vi "Init AC Source.vi"(7 "Trigger frequency  (Hz)":dbl, 8 "error in (no error)":errorcluster, 11 "AC source":T1={"AC Source type"=enum."Agilent 331xxA to 332xxA", "awg lib session"={"type"=enum."Agilent 331xxA to 332xxA", "VISA"="", "enable 10MHz ref"=FALSE, "cmi ckd2"={"VISA"="", "clock source"=enum."Auto", "manual ref clk"=FALSE, "ref clock [Hz]"=0.0, "div mode"=enum."Set divisor directly"}, "cmi sync v3"={"VISA"="", "baud rate [bd/s]"=115200, "source"=enum."Auto", "hv range"=enum."1kV", "fsrc is fixed"=FALSE, "fsrc [Hz]"=10000000.0, "freq integ [s]"=1.0, "freq filter"=5, "trig level"=enum."TTL 5V", "chn1 mode"=enum."Source divider", "chn1 level"=enum."Positive 5V", "chn2 mode"=enum."Source divider", "chn2 level"=enum."Positive 5V", "chn2 div"=1, "chn3 mode"=enum."Chn 1 Active", "chn3 level"=enum."Positive 5V", "chn1 div entry"=enum."Calculate nearest divisor from measured fx", "chn1 dev limit [%]"=1.0, "chn1 check dev"=FALSE}, "trigger"={"source"=enum."Immediate", "level [V]"=0.0, "coupling"=enum."DC", "slope"=enum."POS"}, "HMF2500 cfg"={"Baud Rate"=9600, "Parity"=0, "Data Bits"=8, "Flow Control"=4}}, "DAQmx Device Name"="PXI2Slot6"} {"awg lib session"."HMF2500 cfg"."Flow Control" items=["None", "XON/XOFF", "RTS/CTS", "XON/XOFF & RTS/CTS", "DTR/DSR", "XON/XOFF & DTR/DSR"]; "awg lib session"."HMF2500 cfg"."Data Bits" items=["7"=7, "8"=8]; "awg lib session"."HMF2500 cfg"."Parity" items=["None", "Odd", "Even", "Mark", "Space"]; "awg lib session"."HMF2500 cfg"."Baud Rate" items=["300"=300, "600"=600, "1200"=1200, "2400"=2400, "4800"=4800, "9600"=9600, "19200"=19200]; "awg lib session"."cmi sync v3"."chn2 div" min=1 max=100000000 step=1; "awg lib session"."cmi sync v3"."fsrc [Hz]" format="%_8p"}) -> (0 "error out":errorcluster, 2 "Init status":string, 3 "AC source out":T1={"AC Source type"=enum."Agilent 331xxA to 332xxA", "awg lib session"={"type"=enum."Agilent 331xxA to 332xxA", "VISA"="", "enable 10MHz ref"=FALSE, "cmi ckd2"={"VISA"="", "clock source"=enum."Auto", "manual ref clk"=FALSE, "ref clock [Hz]"=0.0, "div mode"=enum."Set divisor directly"}, "cmi sync v3"={"VISA"="", "baud rate [bd/s]"=115200, "source"=enum."Auto", "hv range"=enum."1kV", "fsrc is fixed"=FALSE, "fsrc [Hz]"=10000000.0, "freq integ [s]"=1.0, "freq filter"=5, "trig level"=enum."TTL 5V", "chn1 mode"=enum."Source divider", "chn1 level"=enum."Positive 5V", "chn2 mode"=enum."Source divider", "chn2 level"=enum."Positive 5V", "chn2 div"=1, "chn3 mode"=enum."Chn 1 Active", "chn3 level"=enum."Positive 5V", "chn1 div entry"=enum."Calculate nearest divisor from measured fx", "chn1 dev limit [%]"=1.0, "chn1 check dev"=FALSE}, "trigger"={"source"=enum."Immediate", "level [V]"=0.0, "coupling"=enum."DC", "slope"=enum."POS"}, "HMF2500 cfg"={"Baud Rate"=9600, "Parity"=0, "Data Bits"=8, "Flow Control"=4}}, "DAQmx Device Name"="PXI2Slot6"} {"awg lib session"."HMF2500 cfg"."Flow Control" items=["None", "XON/XOFF", "RTS/CTS", "XON/XOFF & RTS/CTS", "DTR/DSR", "XON/XOFF & DTR/DSR"]; "awg lib session"."HMF2500 cfg"."Data Bits" items=["7"=7, "8"=8]; "awg lib session"."HMF2500 cfg"."Parity" items=["None", "Odd", "Even", "Mark", "Space"]; "awg lib session"."HMF2500 cfg"."Baud Rate" items=["300"=300, "600"=600, "1200"=1200, "2400"=2400, "4800"=4800, "9600"=9600, "19200"=19200]; "awg lib session"."cmi sync v3"."chn2 div" min=1 max=100000000 step=1; "awg lib session"."cmi sync v3"."fsrc [Hz]" format="%_8p"})   [LabVIEW 2020]
uses:
  Type definitions/AC Source.ctl
  Type definitions/AC Source type.ctl
  external libraries/AWG/AWG Session.ctl
  external libraries/AWG/AWG Type.ctl
  external libraries/AWG/CMI Clock Divider v2/CMI ckd2 Session.ctl
  external libraries/AWG/CMI Clock Divider v2/CMI ckd2 Source Mode.ctl
  external libraries/AWG/CMI Clock Divider v2/CMI ckd2 Divisor Mode.ctl
  external libraries/AWG/CMI Sync V3/CMI Sync V3 session.ctl
  external libraries/AWG/CMI Sync V3/Configure/CMI Sync V3 Reference Clock Source.ctl
  external libraries/AWG/CMI Sync V3/Configure/CMI Sync V3 HV input Range.ctl
  external libraries/AWG/CMI Sync V3/Configure/CMI Sync V3 Trigger Input Level.ctl
  external libraries/AWG/CMI Sync V3/Configure/CMI Sync V3 Channel 1 Mode.ctl
  external libraries/AWG/CMI Sync V3/Configure/CMI Sync V3 Channel Output Levels.ctl
  external libraries/AWG/CMI Sync V3/Configure/CMI Sync V3 Channel 2 Mode.ctl
  external libraries/AWG/CMI Sync V3/Configure/CMI Sync V3 Channel 3 Mode.ctl
  external libraries/AWG/CMI Sync V3/Configure/CMI Sync V3 Channel 1 Divisor Entry Mode.ctl
  external libraries/externals needed for AWG/ADC Trig Config.ctl
  external libraries/externals needed for AWG/ADC Trig Mode Source.ctl
  external libraries/externals needed for AWG/ADC Trig Coupling.ctl
  external libraries/externals needed for AWG/ADC Trig Slope.ctl
  external libraries/AWG/RaS HMF2500/HMF2500 Config.ctl
  external libraries/AWG/AWG.lvlib
  external libraries/Fluke 5XXX Series Multicalibrator/Fluke 5XXX Series Multicalibrators.lvlib
  external libraries/AWG/CMI Sync V3/CMI Sync Unit V3.lvlib
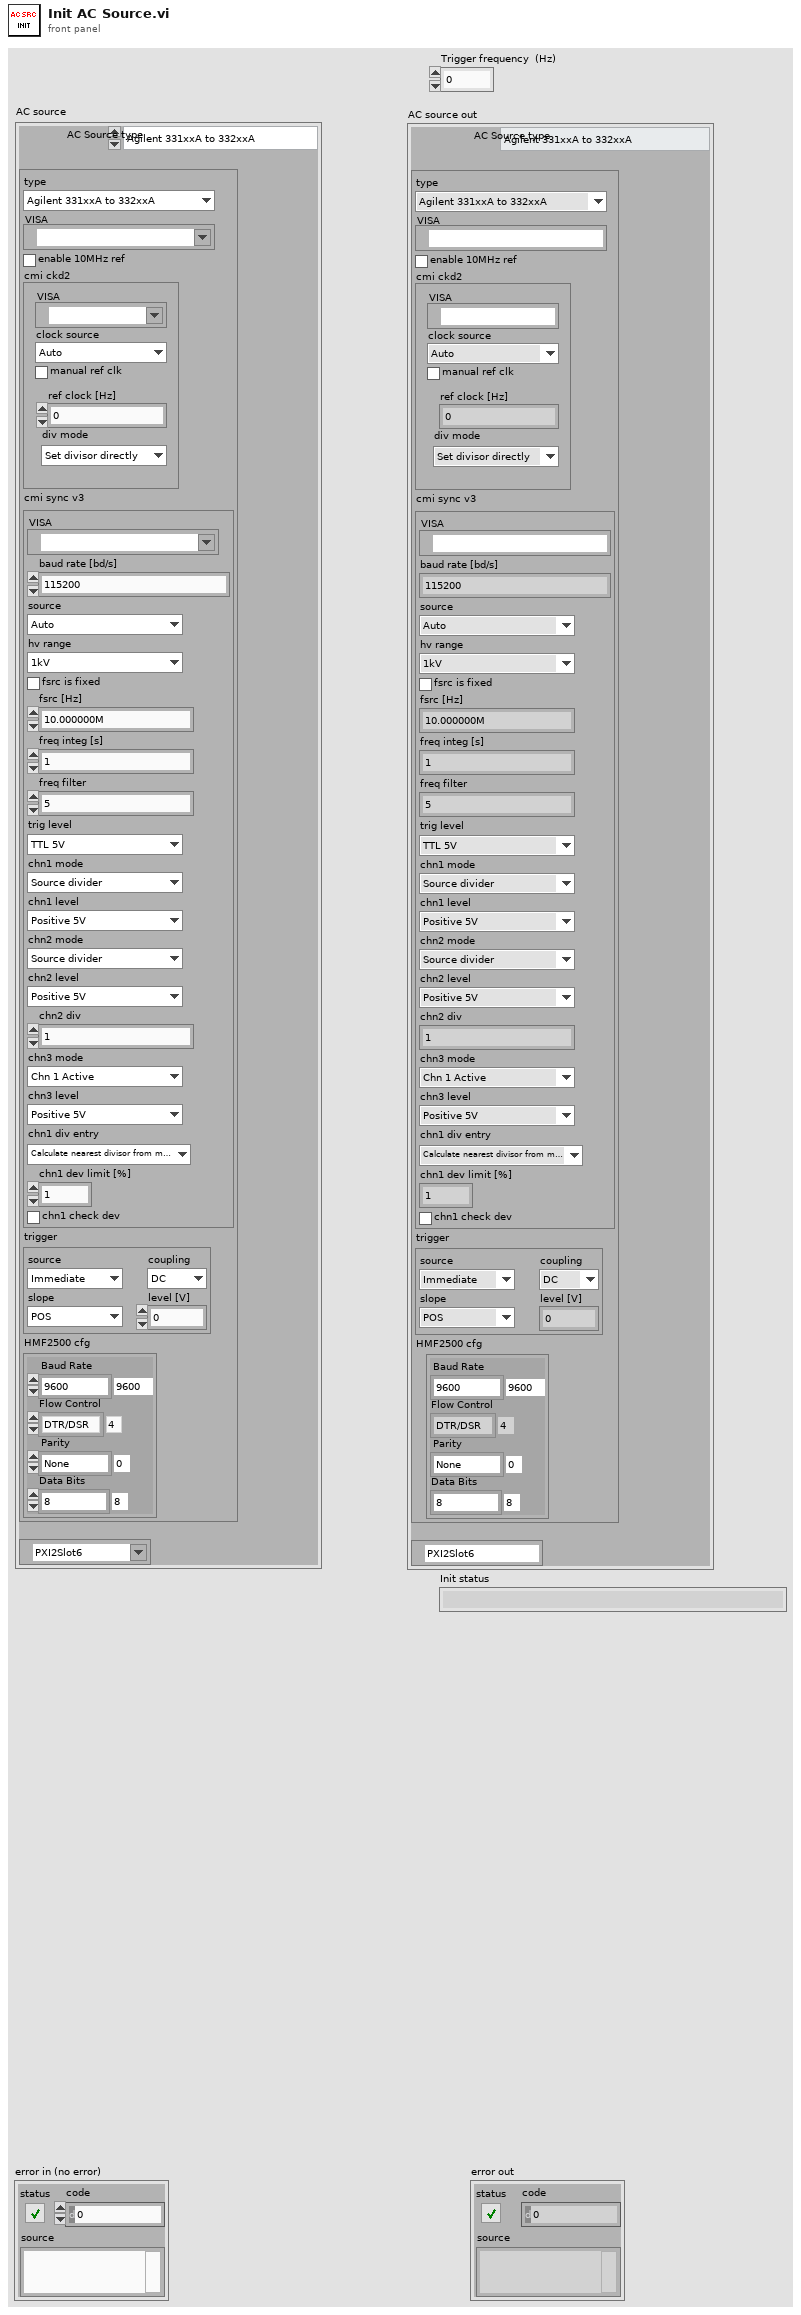
[diagram p1: front panel]
types:
  T1 = typedef "AC Source.ctl" = cluster{"AC Source type":T2, "awg lib session":T3, "DAQmx Device Name":tag}
  T2 = typedef "AC Source type.ctl" = enum16{"Agilent 331xxA to 332xxA", "Agilent 335xxA to 336xxA", "Tektronix AFG3101C", "R&S HMF25xx", "CMI Clock Divider v2", "CMI Sync Unit V3", "NI DAQ", "Fluke 5XXX calibrator", "dummy"}
  T3 = typedef "AWG.lvlib/AWG Session.ctl" = cluster{"type":T4, "VISA":refnum<visa-resource-name>, "enable 10MHz ref":bool, "cmi ckd2":T5, "cmi sync v3":T8, "trigger":T17, "HMF2500 cfg":T21}
  T4 = typedef "AWG.lvlib/AWG Type.ctl" = enum16{"Agilent 331xxA to 332xxA", "Agilent 335xxA to 336xxA", "Tektronix AFG3101C", "R&S HMF25xx", "CMI Clock Divider v2", "CMI Sync Unit V3", "dummy"}
  T5 = typedef "AWG.lvlib/CMI ckd2 Session.ctl" = cluster{"VISA":refnum<visa-resource-name>, "clock source":T6, "manual ref clk":bool, "ref clock [Hz]":dbl, "div mode":T7}
  T6 = typedef "AWG.lvlib/CMI ckd2 Source Mode.ctl" = enum16{"Auto", "LF clock", "HF clock", "Internal"}
  T7 = typedef "AWG.lvlib/CMI ckd2 Divisor Mode.ctl" = enum16{"Set divisor directly", "Set divisor by frequency"}
  T8 = typedef "AWG.lvlib/CMI Sync Unit V3.lvlib/CMI Sync V3 session.ctl" = cluster{"VISA":refnum<visa-resource-name>, "baud rate [bd/s]":i32, "source":T9, "hv range":T10, "fsrc is fixed":bool, "fsrc [Hz]":dbl, "freq integ [s]":dbl, "freq filter":i32, "trig level":T11, "chn1 mode":T12, "chn1 level":T13, "chn2 mode":T14, "chn2 level":T13, "chn2 div":i32, "chn3 mode":T15, "chn3 level":T13, "chn1 div entry":T16, "chn1 dev limit [%]":dbl, "chn1 check dev":bool}
  T9 = typedef "AWG.lvlib/CMI Sync Unit V3.lvlib/CMI Sync V3 Reference Clock Source.ctl" = enum16{"Auto", "Internal", "Logic", "Sine", "HV"}
  T10 = typedef "AWG.lvlib/CMI Sync Unit V3.lvlib/CMI Sync V3 HV input Range.ctl" = enum16{"10V", "60V", "250V", "1kV"}
  T11 = typedef "AWG.lvlib/CMI Sync Unit V3.lvlib/CMI Sync V3 Trigger Input Level.ctl" = enum16{"LVCMOS 3V3", "TTL 5V"}
  T12 = typedef "AWG.lvlib/CMI Sync Unit V3.lvlib/CMI Sync V3 Channel 1 Mode.ctl" = enum16{"Source divider", "DDS absolute", "DDS ratio", "DDS ratio M/N"}
  T13 = typedef "AWG.lvlib/CMI Sync Unit V3.lvlib/CMI Sync V3 Channel Output Levels.ctl" = enum16{"Positive 3V3", "Negative 3V3", "Positive 5V", "Negative 5V"}
  T14 = typedef "AWG.lvlib/CMI Sync Unit V3.lvlib/CMI Sync V3 Channel 2 Mode.ctl" = enum16{"Source divider", "Chn 1 divide"}
  T15 = typedef "AWG.lvlib/CMI Sync Unit V3.lvlib/CMI Sync V3 Channel 3 Mode.ctl" = enum16{"Chn 1 Active", "Chn 2 Active", "Chn 1 Trigger", "Chn 2 Trigger", "Gate", "PPS", "10MHz"}
  T16 = typedef "AWG.lvlib/CMI Sync Unit V3.lvlib/CMI Sync V3 Channel 1 Divisor Entry Mode.ctl" = enum16{"Set divisor directly", "Calculate nearest divisor from measured fx"}
  T17 = typedef "ADC Trig Config.ctl" = cluster{"source":T18, "level [V]":dbl, "coupling":T19, "slope":T20}
  T18 = typedef "ADC Trig Mode Source.ctl" = enum16{"Immediate", "External", "Level"}
  T19 = typedef "ADC Trig Coupling.ctl" = enum16{"DC", "AC"}
  T20 = typedef "ADC Trig Slope.ctl" = enum16{"POS", "NEG"}
  T21 = typedef "AWG.lvlib/HMF2500 Config.ctl" = cluster{"Baud Rate":u32, "Parity":u16, "Data Bits":u16, "Flow Control":u16}
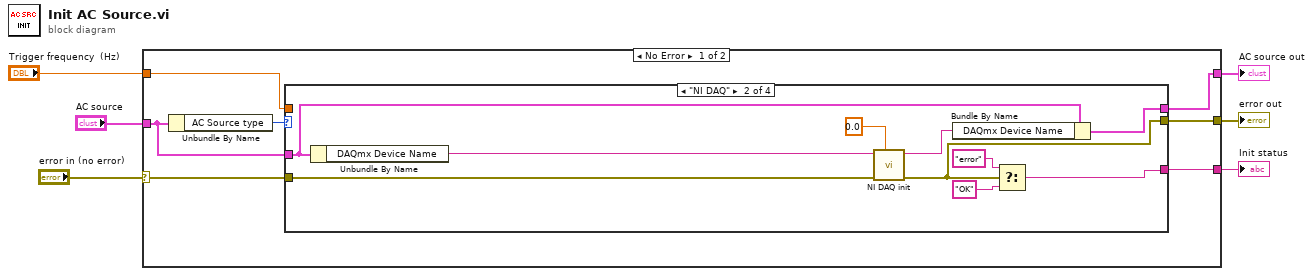
[diagram p0: block diagram]
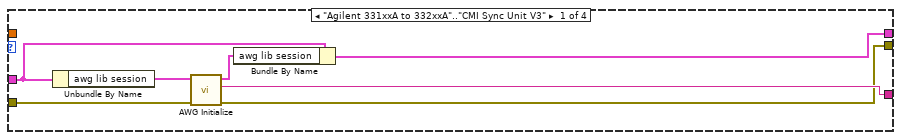
[diagram p2: hidden frame]
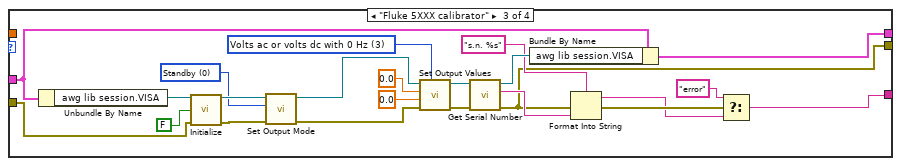
[diagram p3: hidden frame]
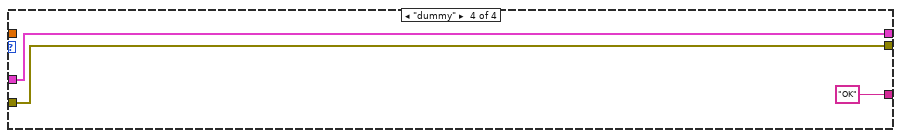
[diagram p4: hidden frame]
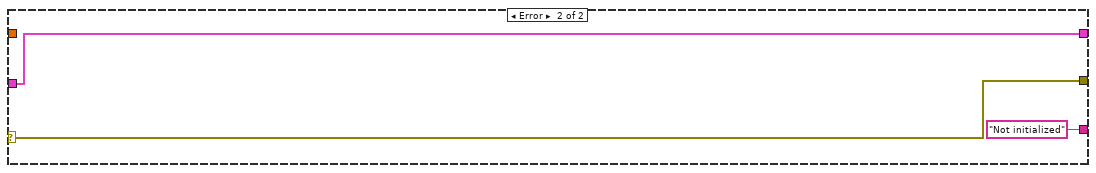
[diagram p5: hidden frame]
diagram:
  n1 = case shown="No Error" "error in (no error)" {
    selector: "error in (no error)" -> [w7 w58]
    tunnel: [w13 w58] -> w6
    tunnel: "AC source" -> [w11 w59]
    tunnel: "Trigger frequency  (Hz)" -> [w10 _]
    tunnel: [w9 w59] -> w3
    tunnel: [w8 "Not initialized" ("idn string")] -> w2
    frame No Error {
      n2 = Unbundle By Name(w11) -> ("AC Source type"=w12:T2)
      n3 = case shown="\"NI DAQ\"" w12 {
        tunnel: w7 -> [w20 w27 w53 w56]
        tunnel: [w15 w25 w33 w56] -> w13
        tunnel: w11 -> [w18 w29 w52 w55]
        tunnel: w10 -> [_ _ _ _]
        tunnel: [w17 w26 w51 w55] -> w9
        tunnel: [w16 w22 w39 "OK" ("idn string")] -> w8
        frame "Agilent 331xxA to 332xxA".."CMI Sync Unit V3" {
          n4 = Unbundle By Name(w18) -> ("awg lib session"=w19:T3)
          n5 = call "AWG Initialize.vi"("error in (no error)"=w20, "awg session in"=w19) -> ("error out"=w15:errorcluster, "idn string"=w16:string, "awg session out"=w14:T3)  [unwired: 7 in]
          n6 = Bundle By Name(cluster=w18, "awg lib session"=w14) -> (w17:T1)
        }
        frame "NI DAQ" {
          n7 = Unbundle By Name(w29) -> ("DAQmx Device Name"=w30:tag)
          n8 = call "NI DAQ init.vi"("trigger frequency"=0.0, "error in"=w27, "DAQmx Device Name"=w30) -> ("error out"=w25:errorcluster, "DAQmx Device Name Out"=w28:tag)  [unwired: 7 in]
          n9 = Bundle By Name(cluster=w29, "DAQmx Device Name"=w28) -> (w26:T1)
          n10 = Select(t="error" ("idn string"), s=w25, f="OK" ("idn string")) -> (s? t:f=w22:string)
        }
        frame "Fluke 5XXX calibrator" {
          w43 = u32 3 items=["Amplitude", "Volts dc or update volts ac", "Volts ac dBm update", "Volts ac or volts dc with 0 Hz", "Volts ac in dBm", "Current dc or update current ac", "Current ac", "Update frequency", "Resistance", "Capacitance", "Temperature (Celsius)", "Temperature (Fahrenheit)", "Power dc or update power ac", "Power ac", "Dual volts dc or update dual ac", "Dual volts ac in volts", "Power ac in dBm update", "Power ac in dBm", "Dual volts ac in dBm update", "Dual volts ac in dBm"] ("Output Value(s) (0 - Amplitude)")
          w44 = u32 0 items=["Standby", "Operate"] ("Output Mode (0: Standby)")
          n11 = Unbundle By Name(w52) -> ("awg lib session.VISA"=w50:refnum<visa-resource-name>)
          n12 = call "Initialize.vi"("VISA resource name"=w50, "Reset (T: Reset)"=FALSE, "error in (no error)"=w53) -> ("VISA resource name out"=w47:refnum<visa-resource-name>, "error out"=w48:errorcluster)  [unwired: 11 in]
          n13 = call "Set Output Mode.vi"("error in (no error)"=w48, "Output Mode (0: Standby)"=w44, "VISA resource name"=w47) -> ("error out"=w46:errorcluster, "VISA resource name out"=w45:refnum<visa-resource-name>)  [unwired: 7 in]
          n14 = call "Set Output Values.vi"("Output Value(s) (0 - Amplitude)"=w43, "error in (no error)"=w46, "Secondary Value (0.0)"=0.0, "Primary Value (0.0)"=0.0, "VISA resource name"=w45) -> ("error out"=w38:errorcluster, "VISA resource name out"=w37:refnum<visa-resource-name>)  [unwired: 5 in]
          n15 = call "Get Serial Number.vi"("error in (no error)"=w38, "VISA resource name"=w37) -> ("error out"=w33:errorcluster, "Serial Number"=w34:string, "VISA resource name out"=w36:refnum<visa-resource-name>)  [unwired: 7 in]
          n16 = Bundle By Name(cluster=w52, "awg lib session.VISA"=w36) -> (w51:T1)
          n17 = Format Into String(format string="s.n. %s", error in=w33, w34) -> (resulting string=w31:string, error out=w32:errorcluster)  [unwired: 1 in]
          n18 = Select(t="error" ("idn string"), s=w32, f=w31) -> (s? t:f=w39:string)
        }
        frame "dummy" {
        }
      }
    }
    frame Error {
    }
  }
  "error out" <- w6
  "AC source out" <- w3
  "Init status" <- w2
